vi "PNT-Data-Write.vi"(0 "Path IN":path, 7 "Data Line":string, 11 "Error IN":errorcluster) -> (4 "Path OUT":path, 15 "Error OUT":errorcluster)   [LabVIEW 2011]
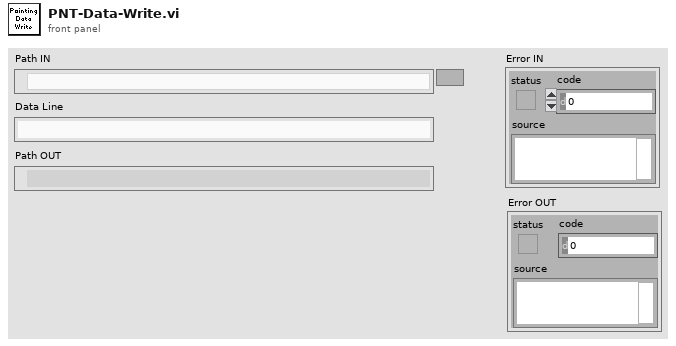
[diagram p1: front panel]
types:
  T1 = enum16{"open", "replace", "create", "open or create", "replace or create", "replace or create with confirmation"}
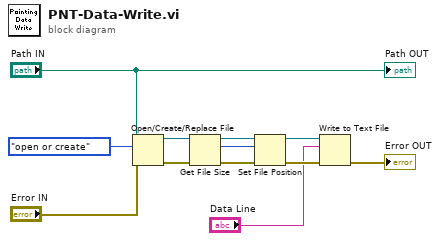
[diagram p0: block diagram]
diagram:
  n1 = Open/Create/Replace File(file path (use dialog)="Path IN", error in="Error IN", operation (0:open)=T1."open or create") -> (refnum out=w9:refnum<file>, error out=w8:errorcluster)  [unwired: 3 in, 1 out]
  n2 = Get File Size(file=w9, error in=w8) -> (refnum out=w10:refnum<file>, size (in bytes)=w5:i64, 0:w7:errorcluster)
  n3 = Set File Position(offset (in bytes) (0)=w5, refnum=w10, error in=w7) -> (refnum out=w11:refnum<file>, error out=w6:errorcluster)  [unwired: 1 in]
  n4 = Write to Text File(file (use dialog)=w11, text="Data Line", error in=w6) -> (error out=→"Error OUT":errorcluster)  [unwired: 1 in, 2 out]
  "Path OUT" <- "Path IN"
